vi "String to Status.vi"(1 "String":string) -> (0 "Result":T1)   [LabVIEW 2020]
uses:
  Controls/PKYK_Status.ctl
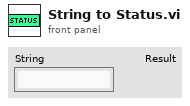
[diagram p1: front panel]
types:
  T1 = typedef "PKYK_Status.ctl" = u16
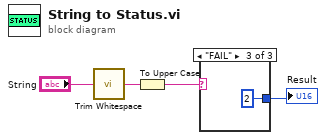
[diagram p0: block diagram]
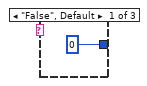
[diagram p2: hidden frame]
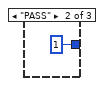
[diagram p3: hidden frame]
diagram:
  n1 = call <vilib>:"Trim Whitespace.vi"("string"="String") -> ("trimmed string"=w1:string)  [unwired: 1 in]
  n2 = To Upper Case(1:w1) -> (0:w2:string)
  n3 = case shown="\"FAIL\"" w2 {
    tunnel: [T1 0 ("Result") T1 1 ("Result") T1 2 ("Result")] -> w4
    frame "False", Default {
    }
    frame "PASS" {
    }
    frame "FAIL" {
    }
  }
  "Result" <- w4
